vi "test pol.vi"() -> ()   [LabVIEW 2019]
uses:
  SubVI/Automation/Automation.lvclass
panel:
  out "x/y":dbl[](array[numeric])
  in  "T_array 2":dbl[](array[numeric])
  out "Number of samples taken":i32
  in  "OK Button 2":bool
  out "error out":errorcluster
  out "Boolean":bool
  out "Last Row":string[](array[string])
  in  "file path (dialog if empty)":path
  in  "stop":bool
  in  "OK Button":bool
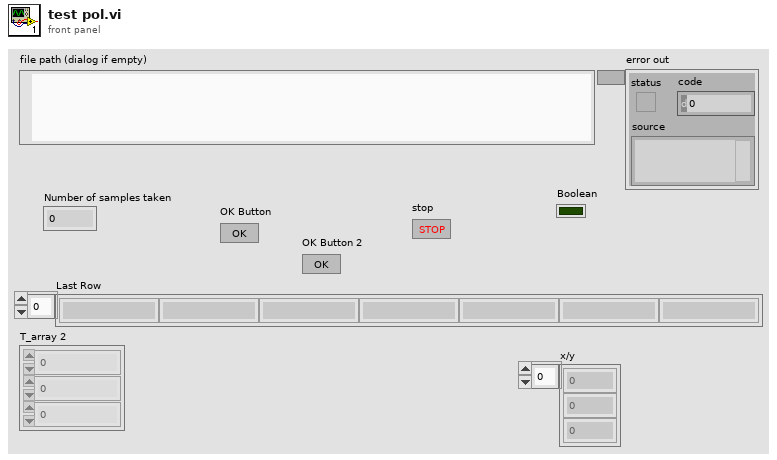
[diagram p1: front panel]
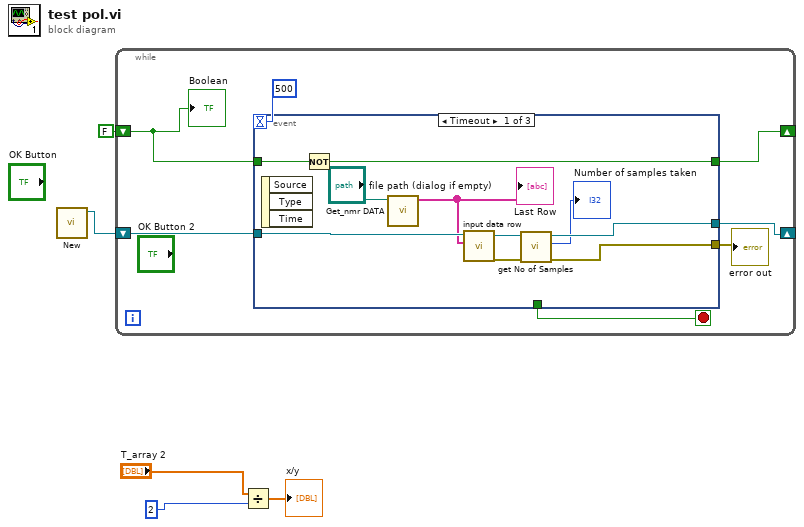
[diagram p0: block diagram]
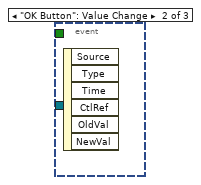
[diagram p2: hidden frame]
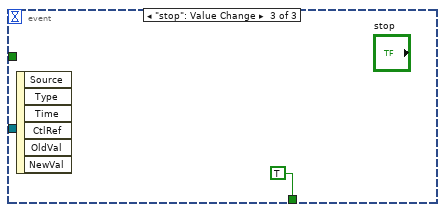
[diagram p3: hidden frame]
diagram:
  n1 = call "New.vi"() -> ("Automation out"=w4:refnum<class "Automation.lvclass">)  [unwired: 10 in, 1 out]
  n2 = while {
    shift-right: [w9] -> _
    shift-left: FALSE ("Boolean") -> [w10]
    shift-right: [w6] -> _
    shift-left: w4 -> [w8]
    stop <- w12 stop-if-true
    n3 = event shown="[0] Timeout" {
      selector: _ -> [_ _ _]
      dyn-events: _ -> [_ _ _]
      timeout: 500 -> [_ _ _]
      tunnel: [_ _ TRUE] -> w12
      tunnel: w10 -> [w22 _ _]
      tunnel: [w21 _ _] -> w9
      tunnel: w8 -> [w20 _ _]
      tunnel: [w15 _ _] -> w7
      tunnel: [w16 _ _] -> w6
      event Timeout {
        n4 = event-data() -> ()  [unwired: 1 in, 3 out]
        n5 = Not(x=w22) -> (.not. x?=w21:bool)
        n6 = call "Get_nmr DATA.vi"("file path (dialog if empty)"="file path (dialog if empty)") -> ("Last Row"=w18:string[])  [unwired: 10 in]
        "Last Row" <- w18
        n7 = call "input data row.vi"("Last row of data file"=w18, "Automation in"=w20) -> ("error out"=w14:errorcluster, "Automation out"=w17:refnum<class "Automation.lvclass">)  [unwired: 5 in, 3 out]
        n8 = call "get No of Samples.vi"("error in (no error)"=w14, "Automation in"=w17) -> ("error out"=w15:errorcluster, "Number of samples taken"=→"Number of samples taken":i32, "Automation out"=w16:refnum<class "Automation.lvclass">)  [unwired: 7 in]
      }
      event "OK Button": Value Change {
        n9 = event-data() -> ()  [unwired: 1 in, 6 out]
      }
      event "stop": Value Change {
        n10 = event-data() -> ()  [unwired: 1 in, 6 out]
      }
    }
    "error out" <- w7
    "Boolean" <- w10
  }
  n11 = Divide(x="T_array 2", y=2) -> (x/y=→"x/y":dbl[])
